vi "multipoint.vi"() -> ()   [LabVIEW 2018]
panel:
  in  "stop":bool
  in  "square":dbl(slide) scale=0.0..40.0
  in  "Slide":dbl(slide) scale=0.0..40.0
  out "Waveform Graph":dynamicdata(graph)
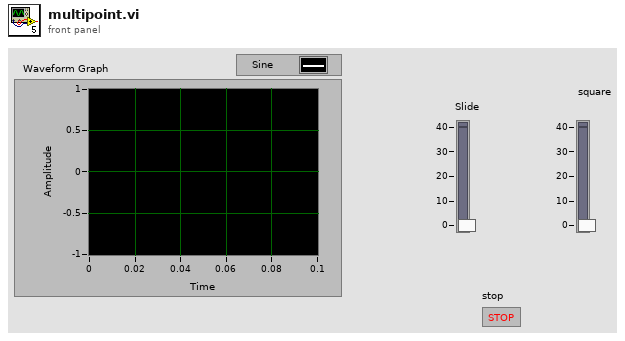
[diagram p1: front panel]
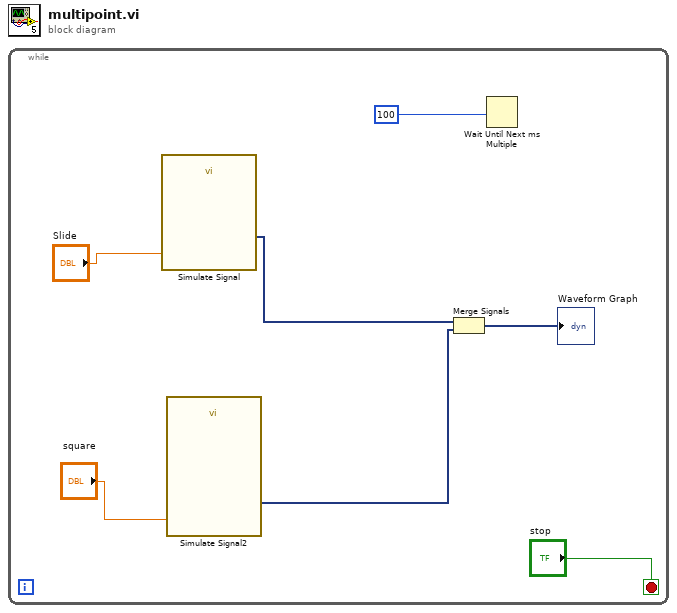
[diagram p0: block diagram]
diagram:
  n1 = while {
    stop <- "stop" stop-if-true
    n2 = call "Simulate Signal"("Frequency"="Slide") -> ("Sine"=w4:dynamicdata)  [unwired: 13 in, 1 out]
    n3 = call "Simulate Signal2"("Frequency"="square") -> ("Square"=w2:dynamicdata)  [unwired: 13 in, 1 out]
    n4 = Merge Signals(w4, w2) -> (→"Waveform Graph":dynamicdata)
    n5 = Wait Until Next ms Multiple(millisecond multiple=100) -> ()  [unwired: 1 out]
  }
